vi "ReadWriteTopicData.vi"(3 "error in (no error)":errorcluster, 4 "timeout ms (1000)":i32=1000, 5 "connection ID in":refnum<k5>) -> (0 "error out":errorcluster, 1 "data out":string, 2 "connection ID out":refnum<k5>)   [LabVIEW 2012]
doc: "Reads and writes topic data"
uses:
  <userlib>/ROS for LabVIEW Software/ROS/MessageParsing/std_msgs/subs/parse_u32_scalar.vi
panel:
  out "received":i32
  out "requested":u32
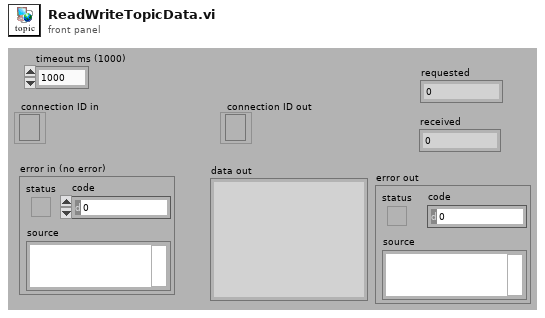
[diagram p1: front panel]
types:
  T1 = enum16{"Standard", "Buffered", "CRLF", "Immediate"}
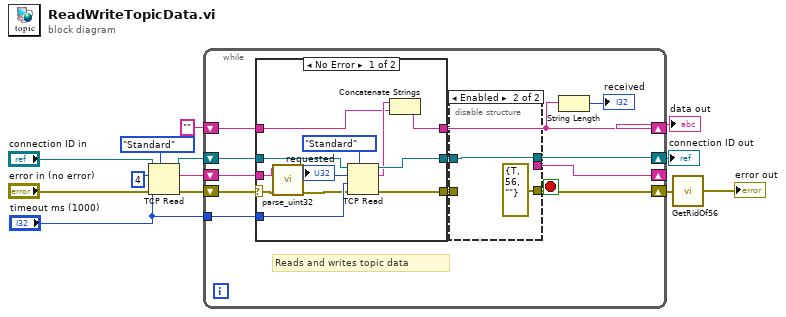
[diagram p0: block diagram]
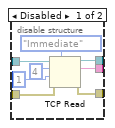
[diagram p2: hidden frame]
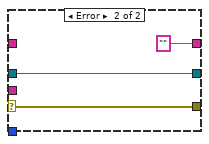
[diagram p3: hidden frame]
diagram:
  n1 = TCP Read(connection ID="connection ID in", bytes to read=4, error in (no error)="error in (no error)", 7:T1."Standard" ("mode (standard)"), 9:"timeout ms (1000)") -> (connection ID out=w10:refnum<k5>, data out=w7:string, error out=w6:errorcluster)
  n2 = while {
    tunnel: "timeout ms (1000)" -> [w22]
    shift-right: [w18] -> _
    shift-left: w7 -> [w24]
    shift-right: [w17] -> w13
    shift-left: w6 -> [w23]
    shift-right: [w20] -> w4
    shift-left: w10 -> [w25]
    shift-right: [w16] -> w2
    shift-left: "" ("data out") -> [w14]
    stop <- w17 stop-if-true
    # "Reads and writes topic data"
    n3 = case shown="No Error" w23 {
      selector: w23 -> [w39 w48]
      tunnel: [w36 "" ("data out")] -> w16
      tunnel: [w47 w48] -> w19
      tunnel: [w46 w50] -> w21
      tunnel: w25 -> [w45 w50]
      tunnel: w24 -> [w40 _]
      tunnel: w22 -> [w43 _]
      tunnel: w14 -> [w37 _]
      frame No Error {
        n4 = call-poly <userlib>:"parse_uint32.vi"("error in"=w39, "msg in"=w40) -> ("error out"=w41:errorcluster, "number"=w42:u32)  [unwired: 3 in, 1 out]
        "requested" <- w42
        n5 = TCP Read(connection ID=w45, bytes to read=w42, error in (no error)=w41, 7:T1."Standard" ("mode (standard)"), 9:w43) -> (connection ID out=w46:refnum<k5>, data out=w38:string, error out=w47:errorcluster)
        n6 = Concatenate Strings(w38, w37) -> (w36:string)
      }
      frame Error {
      }
    }
    n7 = disable-structure shown="Enabled" {
      disable-tunnel: w21 -> [w33 w35]
      disable-tunnel: [w30 w35] -> w20
      disable-tunnel: w19 -> [w29 _]
      disable-tunnel: [w28 _] -> w18
      disable-tunnel: [w26 errorcluster {"status"=TRUE, "code"=56, "source"=""} ("error out")] -> w17
      frame Disabled {
        n8 = TCP Read(connection ID=w33, bytes to read=4, error in (no error)=w29, 7:T1."Immediate" ("mode (standard)"), 9:1 ("timeout ms (25000)")) -> (connection ID out=w30:refnum<k5>, data out=w28:string, error out=w26:errorcluster)
      }
      frame Enabled {
      }
    }
    n9 = String Length(string=w16) -> (length=→"received":i32)
  }
  "data out" <- w2
  "connection ID out" <- w4
  n10 = call <userlib>:"GetRidOf56.vi"("error in (no error)"=w13) -> ("error out"=→"error out":errorcluster)
